vi "PrcoessStepFocus.vi"(8 "Error In":errorcluster, 10 "AllProcessSettingOut":T1[](array[typedef]), 11 "MulticolumnListbox in":refnum<vi>) -> (0 "Error Out":errorcluster)   [LabVIEW 2019]
uses:
  Controls/Process_Setting.ctl
  Ctrl/VisionProcessName.ctl
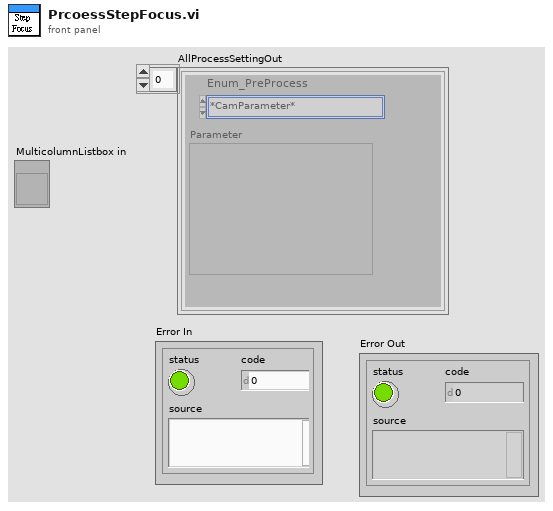
[diagram p1: front panel]
types:
  T1 = typedef "Process_Setting.ctl" = cluster{"Enum_PreProcess":T2, "Parameter":string}
  T2 = typedef "VisionProcessName.ctl" = enum16{"*CamParameter*", "CamAttributes", "*Preprocess*", "CG_Brightness", "C_Plane Extraction", "C_Threshold", "G_Lookup Table", "G_Threshold"}
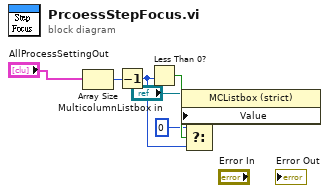
[diagram p0: block diagram]
diagram:
  n1 = Array Size(array="AllProcessSettingOut") -> (size(s)=w7:i32)
  n2 = Decrement(x=w7) -> (x-1=w5:i32)
  n3 = Less Than 0?(x=w5) -> (x < 0?=w6:bool)
  n4 = Select(t=0, s=w6, f=w5) -> (s? t:f=w3:i32)
  n5 = property on="Property Node" class="MCListbox (strict)"(reference="MulticolumnListbox in", "Value"=w3) -> ()  [unwired: 1 in, 2 out]
